vi "Core Actor - Close User Events.vi"(8 "error in (no error)":errorcluster, 11 "Child_1_Class in":refnum<class "GUI_Class.lvclass">) -> (0 "error out":errorcluster, 3 "Child_1_Class out":refnum<class "GUI_Class.lvclass">)   [LabVIEW 2023, in "GUI_Actor.lvlib" / "GUI_Class.lvclass"]
uses:
  GUI_Class.lvclass
  Usr Ev/GUI - Ctrl - Action.ctl
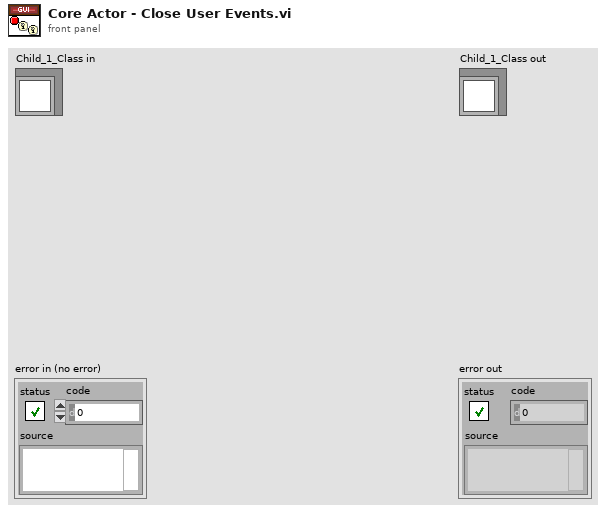
[diagram p1: front panel]
types:
  T1 = typedef "GUI_Actor.lvlib/GUI_Class.lvclass/GUI - Ctrl - Action.ctl" = enum16{"Reg Ev", "Get Refs", "Close Ev", "Populate Enum with Events"}
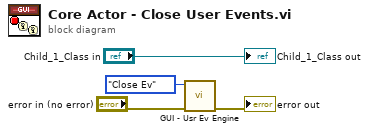
[diagram p0: block diagram]
diagram:
  n1 = call "GUI - Usr Ev Engine.vi"("error in (no error)"="error in (no error)", "Action"=GUI_-_Ctrl_-_Action."Close Ev") -> ("error out"=→"error out":errorcluster)  [unwired: 6 in, 3 out]
  "Child_1_Class out" <- "Child_1_Class in"
